vi "LSX Get Encoder Ref Signal.vi"(0 "lLSID":i32, 1 "plRR":i32, 5 "plXR":i32, 7 "plYR":i32, 9 "plZR":i32, 11 "error in (no error)":errorcluster) -> (3 "plRR out":i32, 4 "function return":i32, 6 "plXR out":i32, 8 "plYR out":i32, 10 "plZR out":i32, 15 "error out":errorcluster)   [LabVIEW 2018, in "Tango.lvlib"]
doc: "TANGOAPI int TANGOCALL LSX_GetEncoderRefSignal (int lLSID, int *plXR, int *plYR, int *plZR, int *plRR);"
uses:
  <userlib>/Tango/Tango.lvlib
  <userlib>/Tango/Tango_DLL.dll
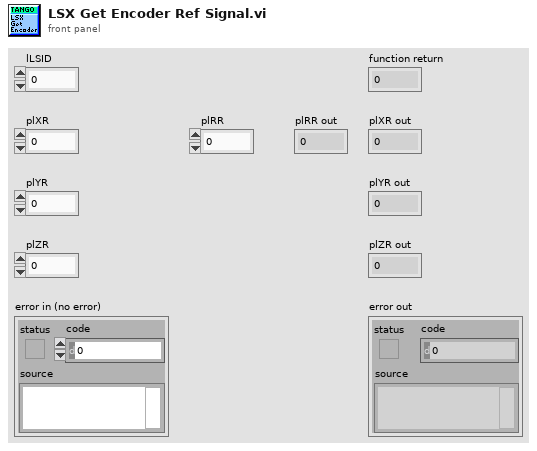
[diagram p1: front panel]
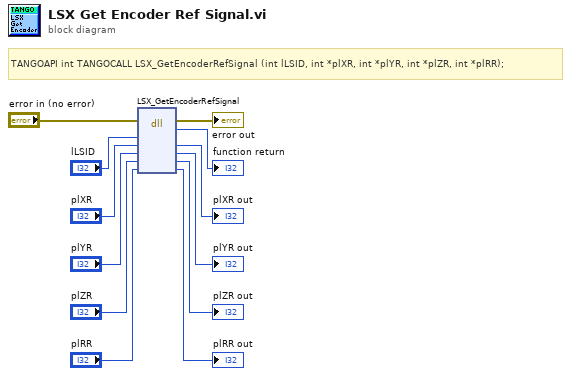
[diagram p0: block diagram]
diagram:
  # "TANGOAPI int TANGOCALL LSX_GetEncoderRefSignal (int lLSID, int *plXR, int *plYR, int *plZR, int *plRR);"
  n1 = dll-call lib="C:/Program Files (x86)/National Instruments/LabVIEW 2018/user.lib/Tango/Tango_DLL.*" fn="LSX_GetEncoderRefSignal"(error in="error in (no error)", "lLSID"="lLSID", "plXR"="plXR", "plYR"="plYR", "plZR"="plZR", "plRR"="plRR") -> (error out=→"error out":errorcluster, →"function return":i32, "plXR"=→"plXR out":i32, "plYR"=→"plYR out":i32, "plZR"=→"plZR out":i32, "plRR"=→"plRR out":i32)  [unwired: 3 in, 1 out]
